vi "Launcher.vi"   [LabVIEW 2020]
uses:
  [MV] Key Generator/[MV] Key Generator/[MV] Key Generator.lvclass
  <vilib>/ActorFramework/Actor/Actor.lvclass
panel:
  # "注册机"
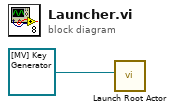
[diagram p0: block diagram]
diagram:
  n1 = call <vilib>:"Launch Root Actor.vi"("Actor"=refnum<class "[MV] Key Generator.lvclass"> refnum ("[MV] Key Generator.lvlib:[MV] Key Generator.lvclass")) -> ()  [unwired: 9 in, 2 out]
